vi "Gripper Control.vi"(1 "Close Gripper":bool, 2 "Gripper Error":errorcluster, 3 "Open Gripper":bool) -> (0 "error out":errorcluster)   [LabVIEW 2014]
uses:
  <vilib>/Rock Robotics/WPI/Solenoid/WPI_SolenoidValue.ctl
  <vilib>/Rock Robotics/WPI/Solenoid/WPI_SolenoidGetEnum.vi
  <vilib>/Rock Robotics/WPI/Solenoid/WPI_SolenoidSetEnum.vi
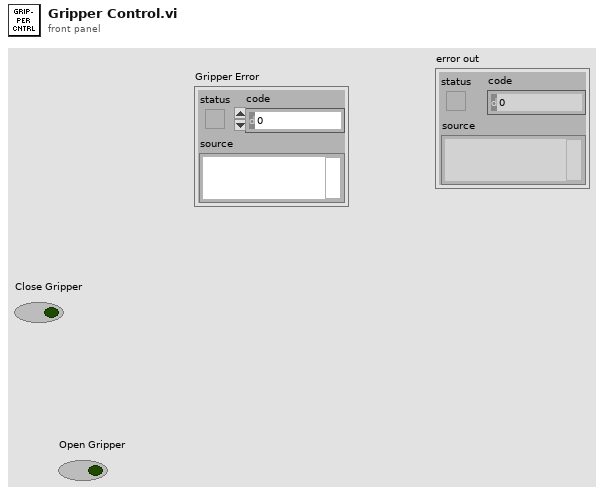
[diagram p1: front panel]
types:
  T1 = typedef "WPI_SolenoidDevRef.ctl" = cluster{"DevStatus":errorcluster, "Pneumatics Control Module":u8, "Forward Solenoid Channel":T2, "Reverse Solenoid Channel":T2}
  T2 = typedef "WPI_SolenoidChannel.ctl" = enum8{"Solenoid 0", "Solenoid 1", "Solenoid 2", "Solenoid 3", "Solenoid 4", "Solenoid 5", "Solenoid 6", "Solenoid 7", "Invalid"}
  T3 = typedef "WPI_SolenoidValue.ctl" = enum16{"Off", "On", "Forward", "Reverse"}
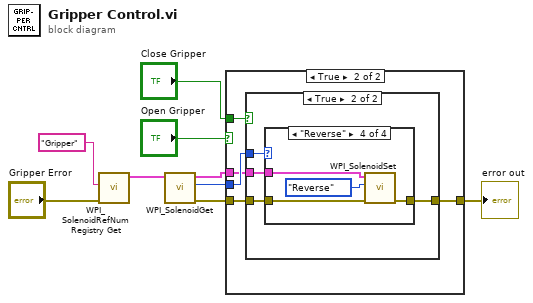
[diagram p0: block diagram]
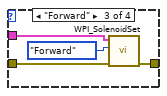
[diagram p4: hidden frame]
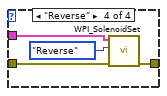
[diagram p5: hidden frame]
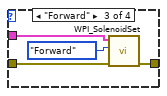
[diagram p8: hidden frame]
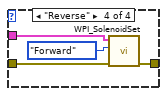
[diagram p9: hidden frame]
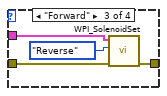
[diagram p12: hidden frame]
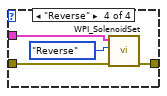
[diagram p13: hidden frame]
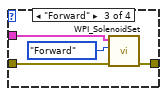
[diagram p16: hidden frame]
diagram:
  n1 = call <vilib>:"WPI_SolenoidRefNum Registry Get.vi"("error in (no error)"="Gripper Error", "refnum name"="Gripper") -> ("SolenoidDevRef"=w9:T1)  [unwired: 8 in, 1 out]
  n2 = call-poly <vilib>:"WPI_SolenoidGet.vi"("SolenoidDevRef"=w9) -> ("error out"=w5:errorcluster, "Value"=w4:T3, "SolenoidDevRef"=w6:T1)  [unwired: 8 in]
  n3 = case shown="True" "Open Gripper" {
    selector: "Open Gripper" -> [w10 _]
    tunnel: "Close Gripper" -> [_ w47]
    tunnel: w4 -> [w12 w46]
    tunnel: w6 -> [w14 w45]
    tunnel: w5 -> [w13 w44]
    tunnel: [w11 w43] -> w1
    frame False {
      n4 = case shown="False" w10 {
        tunnel: w12 -> [w18 w32]
        tunnel: w14 -> [w17 w31]
        tunnel: w13 -> [w16 w30]
        tunnel: [w15 w29] -> w11
        frame False {
          n5 = case shown="\"Off\", Default" w18 {
            tunnel: w17 -> [_ _ w24 w27]
            tunnel: w16 -> [w19 w20 w22 w26]
            tunnel: [w19 w20 w21 w25] -> w15
            frame "Off", Default {
            }
            frame "On" {
            }
            frame "Forward" {
              n6 = call-poly <vilib>:"WPI_SolenoidSet.vi"("error in (no error)"=w22, "Value"=WPI_SolenoidValue."Forward", "SolenoidDevRef"=w24) -> ("error out"=w21:errorcluster)  [unwired: 7 in, 1 out]
            }
            frame "Reverse" {
              n7 = call-poly <vilib>:"WPI_SolenoidSet.vi"("error in (no error)"=w26, "Value"=WPI_SolenoidValue."Reverse", "SolenoidDevRef"=w27) -> ("error out"=w25:errorcluster)  [unwired: 7 in, 1 out]
            }
          }
        }
        frame True {
          n8 = case shown="\"Off\", Default" w32 {
            tunnel: w31 -> [_ _ w38 w41]
            tunnel: w30 -> [w33 w34 w36 w40]
            tunnel: [w33 w34 w35 w39] -> w29
            frame "Off", Default {
            }
            frame "On" {
            }
            frame "Forward" {
              n9 = call-poly <vilib>:"WPI_SolenoidSet.vi"("error in (no error)"=w36, "Value"=WPI_SolenoidValue."Forward", "SolenoidDevRef"=w38) -> ("error out"=w35:errorcluster)  [unwired: 7 in, 1 out]
            }
            frame "Reverse" {
              n10 = call-poly <vilib>:"WPI_SolenoidSet.vi"("error in (no error)"=w40, "Value"=WPI_SolenoidValue."Forward", "SolenoidDevRef"=w41) -> ("error out"=w39:errorcluster)  [unwired: 7 in, 1 out]
            }
          }
        }
      }
    }
    frame True {
      n11 = case shown="True" w47 {
        tunnel: w46 -> [w51 w65]
        tunnel: w45 -> [w50 w64]
        tunnel: w44 -> [w49 w63]
        tunnel: [w48 w62] -> w43
        frame False {
          n12 = case shown="\"Off\", Default" w51 {
            tunnel: w50 -> [_ _ w57 w60]
            tunnel: w49 -> [w52 w53 w55 w59]
            tunnel: [w52 w53 w54 w58] -> w48
            frame "Off", Default {
            }
            frame "On" {
            }
            frame "Forward" {
              n13 = call-poly <vilib>:"WPI_SolenoidSet.vi"("error in (no error)"=w55, "Value"=WPI_SolenoidValue."Reverse", "SolenoidDevRef"=w57) -> ("error out"=w54:errorcluster)  [unwired: 7 in, 1 out]
            }
            frame "Reverse" {
              n14 = call-poly <vilib>:"WPI_SolenoidSet.vi"("error in (no error)"=w59, "Value"=WPI_SolenoidValue."Reverse", "SolenoidDevRef"=w60) -> ("error out"=w58:errorcluster)  [unwired: 7 in, 1 out]
            }
          }
        }
        frame True {
          n15 = case shown="\"Reverse\"" w65 {
            tunnel: w64 -> [_ _ w71 w74]
            tunnel: w63 -> [w66 w67 w69 w73]
            tunnel: [w66 w67 w68 w72] -> w62
            frame "Off", Default {
            }
            frame "On" {
            }
            frame "Forward" {
              n16 = call-poly <vilib>:"WPI_SolenoidSet.vi"("error in (no error)"=w69, "Value"=WPI_SolenoidValue."Forward", "SolenoidDevRef"=w71) -> ("error out"=w68:errorcluster)  [unwired: 7 in, 1 out]
            }
            frame "Reverse" {
              n17 = call-poly <vilib>:"WPI_SolenoidSet.vi"("error in (no error)"=w73, "Value"=WPI_SolenoidValue."Reverse", "SolenoidDevRef"=w74) -> ("error out"=w72:errorcluster)  [unwired: 7 in, 1 out]
            }
          }
        }
      }
    }
  }
  "error out" <- w1
